vi "IMS Stepper Read Position.vi"(0 "Instrument Address":refnum<visa-resource-name>, 1 "Motor Number":u32=1 min=1 max=255 step=1, 2 "error in (no error)":errorcluster) -> (3 "Instrument Address Out":refnum<visa-resource-name>, 4 "Response":dbl format="%.4f", 6 "error out":errorcluster)   [LabVIEW 2025]
doc: "Author: Scott Hannahs <sth@magnet.fsu.edu>\n\nThis software is licensed for use under the “MIT License\"\nCopyright (c) 2025 Scott Hannahs, sth@sth@magnet.sthnet.net\n\nPermission is hereby granted, free of charge, to any person obtaining a copy of this software and associated documentation files (the \"Software\"), to deal in the Software without restriction, including without limitation the rights to use, copy, modify, merge, publish, distribute, sublicense, and/or sell copies of the Software, and to permit persons to whom the Software is furnished to do so, subject to the following conditions: The above copyright notice and this permission notice shall be included in all copies or substantial portions of the Software.\n\nTHE SOFTWARE IS PROVIDED \"AS IS\", WITHOUT WARRANTY OF ANY KIND, EXPRESS OR IMPLIED, INCLUDING BUT NOT LIMITED TO THE WARRANTIES OF MERCHANTABILITY, FITNESS FOR A PARTICULAR PURPOSE AND NONINFRINGEMENT. IN NO EVENT SHALL THE AUTHORS OR COPYRIGHT HOLDERS BE LIABLE FOR ANY CLAIM, DAMAGES OR OTHER LIABILITY, WHETHER IN AN ACTION OF CONTRACT, TORT OR OTHERWISE, ARISING FROM, OUT OF OR IN CONNECTION WITH THE SOFTWARE OR THE USE OR OTHER DEALINGS IN THE SOFTWARE."
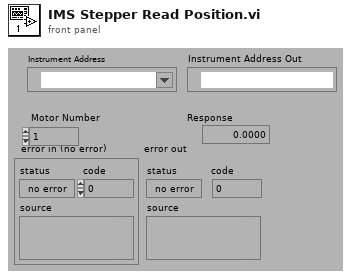
[diagram p1: front panel]
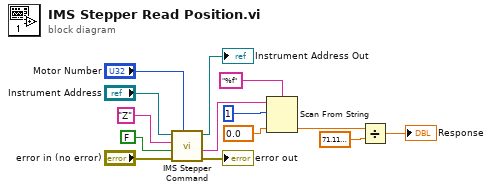
[diagram p0: block diagram]
diagram:
  n1 = call "IMS Stepper Command.vi"("Motor Number"="Motor Number", "error in (no error)"="error in (no error)", "Mode"=FALSE, "Command"="Z", "Instrument Address"="Instrument Address") -> ("error out"=→"error out":errorcluster, "Response"=w7:string, "Instrument Address Out"=→"Instrument Address Out":refnum<visa-resource-name>)  [unwired: 1 in, 1 out]
  n2 = Scan From String(format string="%f", input string=w7, initial scan location=u32 1, default 1=0.0 ("default value 1")) -> (output 1=w9:dbl)  [unwired: 1 in, 3 out]
  n3 = Divide(x=w9, y=71.111111) -> (x/y=→"Response":dbl)
